vi "Calculate.vi"(8 "error in (no error)":errorcluster, 9 "Operand 2":dbl, 10 "Operand 1":dbl, 11 "Addition in":refnum<class "Multiply.lvclass">) -> (0 "error out":errorcluster, 3 "Addition out":refnum<class "Multiply.lvclass">)   [LabVIEW 2013, in "Operators.lvlib" / "Multiply.lvclass"]
uses:
  Multiply.lvclass
  Multiply.lvclass/Multiply.ctl
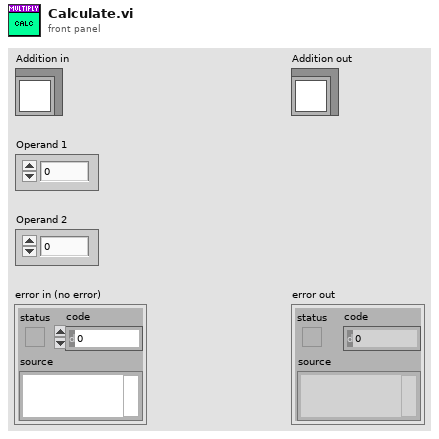
[diagram p1: front panel]
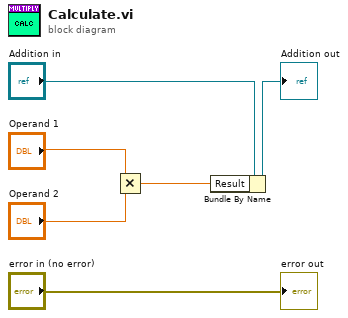
[diagram p0: block diagram]
diagram:
  n1 = Multiply(x="Operand 1", y="Operand 2") -> (x*y=w1:dbl)
  n2 = Bundle By Name(cluster="Addition in", "Result"=w1) -> (→"Addition out":refnum<class "Multiply.lvclass">)
  "error out" <- "error in (no error)"
